vi "hEnable.vi"(7 "LabVIEW Web Service Request":refnum<class "Web Request.lvclass">, 10 "hID":string, 11 "Val":u8) -> ()   [LabVIEW 2014]
uses:
  <vilib>/wsapi/Web Request.lvclass
  Controller/Controller.lvclass
  reusable/Session APIs/CVT/CVT.lvclass
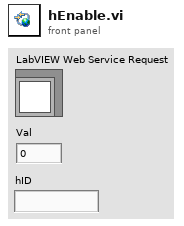
[diagram p1: front panel]
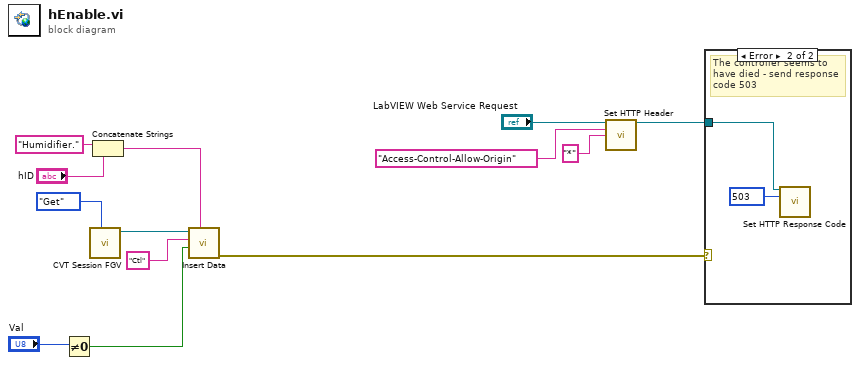
[diagram p0: block diagram]
diagram:
  n1 = Not Equal To 0?(x="Val") -> (x != 0?=w1:bool)
  n2 = call "CVT Session FGV.vi"("State"=enum16{"Init", "Get"}."Get") -> ("CVT Session Out"=w9:refnum<data-value>)  [unwired: 10 in]
  n3 = Concatenate Strings("Humidifier." ("string"), "hID") -> (w4:string)
  n4 = call "Insert Data.vi"("Group"=w4, "Data"=w1, "tag"="Ctl", "CVT Session In"=w9) -> ("error out"=w5:errorcluster)  [unwired: 6 in, 1 out]
  n5 = call <vilib>:"Set HTTP Header.vi"("LabVIEW Web Service Request"="LabVIEW Web Service Request", "header"="Access-Control-Allow-Origin", "header value"="*") -> ("LabVIEW Web Service Request out"=w11:refnum<class "Web Request.lvclass">)  [unwired: 11 in, 1 out]
  n6 = case shown="Error" w5 {
    tunnel: w11 -> [_ w14]
    frame No Error {
    }
    frame Error {
      w15 = 503 items=["100"=100, "101"=101, "200"=200, "201"=201, "202"=202, "203"=203, "204"=204, "205"=205, "206"=206, "300"=300, "301"=301, "302"=302, "303"=303, "304"=304, "305"=305, "306"=306, "307"=307, "400"=400, "401"=401, "402"=402, "403"=403, "404"=404, "405"=405, "406"=406, "407"=407, "408"=408, "409"=409, "410"=410, "411"=411, "412"=412, "413"=413, "414"=414, "415"=415, "416"=416, "417"=417, "500"=500, "501"=501, "502"=502, "503"=503, "504"=504, "505"=505] ("response code (200)")
      # "The controller seems to have died - send response code 503"
      n7 = call <vilib>:"Set HTTP Response Code.vi"("LabVIEW Web Service Request"=w14, "response code (200)"=w15) -> ()  [unwired: 12 in, 2 out]
    }
  }
